vi "ReverseDataI8.vi"(1 "Array in":i8[][](array[numeric])) -> (0 "Array out":i8[][](array[numeric]))   [LabVIEW 2022 SP3]
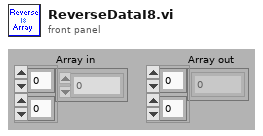
[diagram p1: front panel]
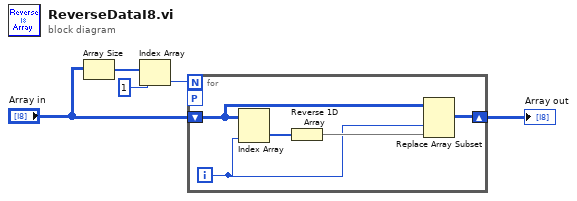
[diagram p0: block diagram]
diagram:
  n1 = Array Size(array="Array in") -> (size(s)=w5:i32[])
  n2 = Index Array(array=w5, index=1) -> (element=w2:i32)
  n3 = for {
    N: w2 -> [_]
    shift-right: [w9] -> w3
    shift-left: "Array in" -> [w8]
    workers-P: _ -> [_]
    i -> [w6]
    n4 = Index Array(array=w8, index (col)=w6) -> (element=w10:i8[])  [unwired: 1 in]
    n5 = Reverse 1D Array(array=w10) -> (reversed array=w7:i8[])
    n6 = Replace Array Subset(array=w8, new element=w7, index (col)=w6) -> (w9:i8[][])  [unwired: 1 in]
  }
  "Array out" <- w3
